vi "wsRegUnregEvents.vi"(8 "Error In":errorcluster, 9 "Event Name (empty =all)":string, 10 "Action":enum16{"Register", "Unregister"}(ring), 11 "References":T1) -> (0 "Error Out":errorcluster, 3 "References Out":T1)   [LabVIEW 2018, in "HASS-LV-WS_integration.lvlib"]
uses:
  HASS-LV-WS_integration.lvlib
  TypeDef/ReferencesTypeDef.ctl
  TypeDef/QueueTypeDef.ctl
  TypeDef/EventTypeDef.ctl
  TypeDef/registeredEventTypeDef.ctl
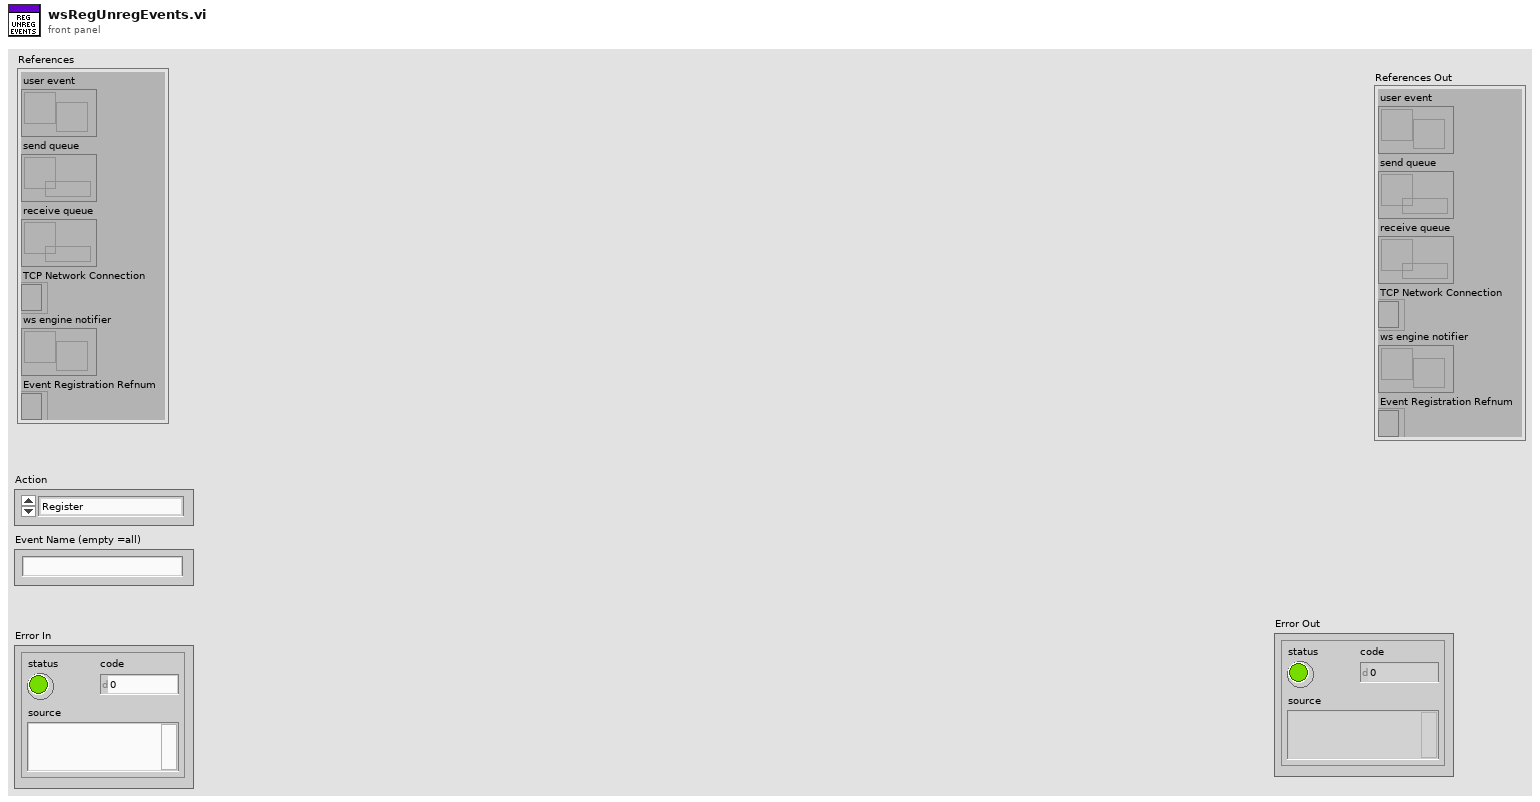
[diagram p1: front panel]
types:
  T1 = typedef "HASS-LV-WS_integration.lvlib/ReferencesTypeDef.ctl" = cluster{"user event":refnum<user-event>, "send queue":refnum<queue>, "receive queue":refnum<queue>, "TCP Network Connection":refnum<k5>, "ws engine notifier ":refnum<notifier>, "Event Registration Refnum":refnum<event-registration>}
  T2 = typedef "HASS-LV-WS_integration.lvlib/EventTypeDef.ctl" = cluster{"Data":variant, "Command":string}
  T3 = typedef "HASS-LV-WS_integration.lvlib/registeredEventTypeDef.ctl" = enum16{"Init", "Register", "Unregister", "Get MSG ID", "Get Event Name", "Get All Events"}
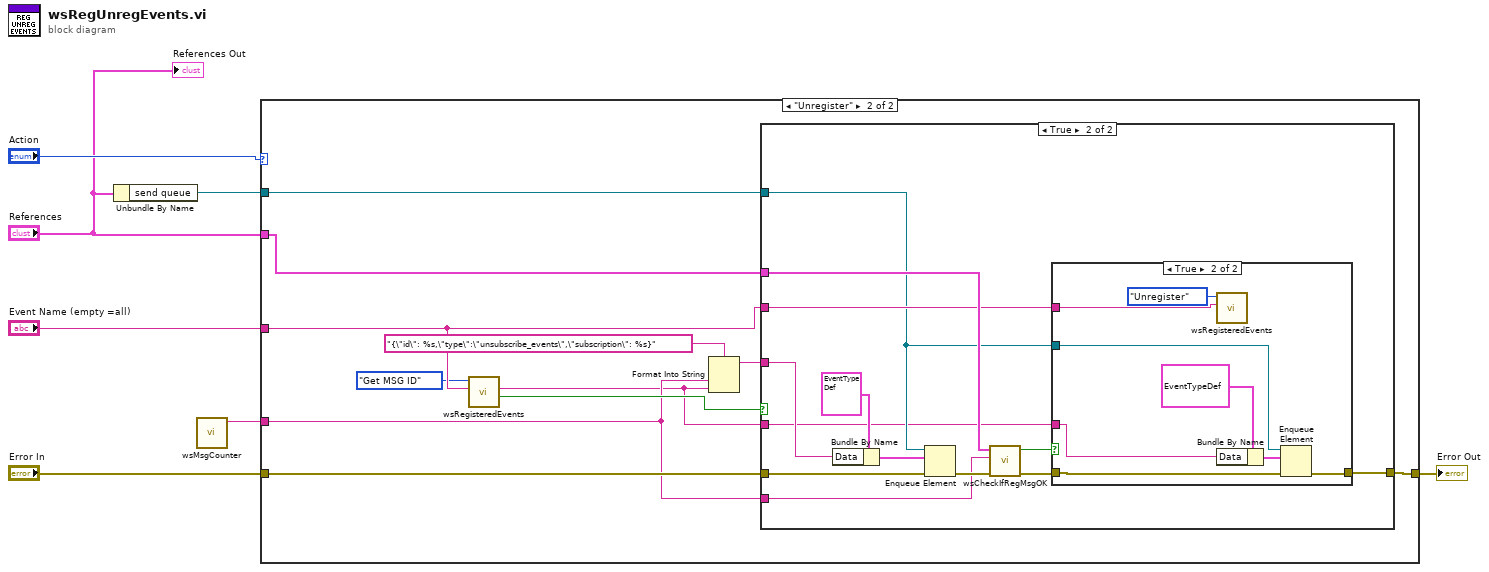
[diagram p0: block diagram]
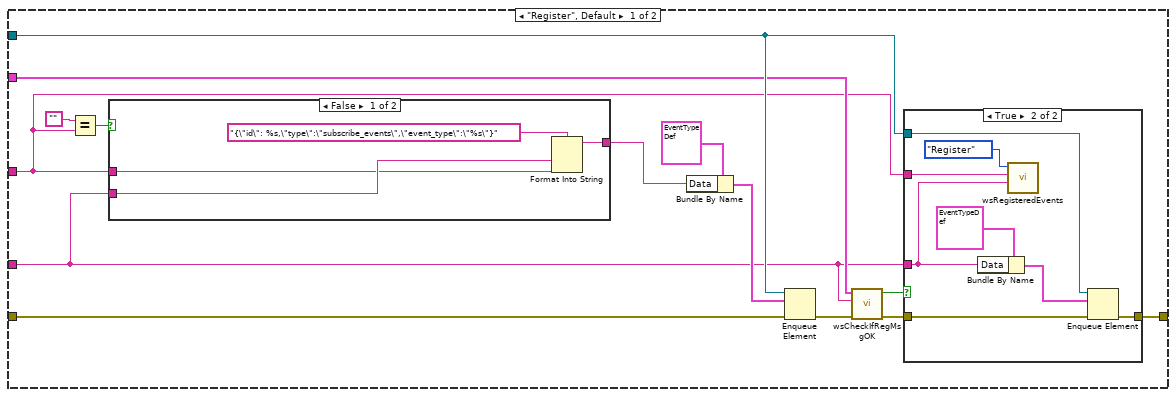
[diagram p2: hidden frame]
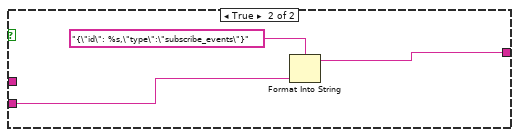
[diagram p4: hidden frame]
diagram:
  n1 = Unbundle By Name("References") -> ("send queue"=w6:refnum<queue>)
  n2 = call "wsMsgCounter.vi"() -> ("msgCounter"=w4:string)  [unwired: 11 in]
  n3 = case shown="\"Unregister\"" "Action" {
    tunnel: "Event Name (empty =all)" -> [w8 w42]
    tunnel: w4 -> [w9 w40]
    tunnel: w6 -> [w13 w46]
    tunnel: "Error In" -> [w16 w45]
    tunnel: "References" -> [w11 w43]
    tunnel: [w10 w41] -> w2
    frame "Register", Default {
      n4 = Equal?(x="", y=w8) -> (x = y?=w20:bool)
      n5 = case shown="False" w20 {
        tunnel: w9 -> [w33 w36]
        tunnel: w8 -> [w32 _]
        tunnel: [w31 w35] -> w17
        frame False {
          n6 = Format Into String(format string="{\"id\": %s,\"type\":\"subscribe_events\",\"event_type\":\"%s\"}", w33, w32) -> (resulting string=w31:string)  [unwired: 2 in, 1 out]
        }
        frame True {
          n7 = Format Into String(format string="{\"id\": %s,\"type\":\"subscribe_events\"}", w36) -> (resulting string=w35:string)  [unwired: 2 in, 1 out]
        }
      }
      n8 = Bundle By Name(cluster=T2 {"Data"=variant, "Command"="Send"} ("element"), "Data"=w17) -> (w18:T2)
      n9 = Enqueue Element(queue=w13, element=w18, error in (no error)=w16) -> (error out=w15:errorcluster)  [unwired: 1 in, 2 out]
      n10 = call "wsCheckIfRegMsgOK.vi"("error in (no error)"=w15, "msgCounter"=w9, "References"=w11) -> ("error out"=w12:errorcluster, "Success?"=w14:bool)  [unwired: 6 in, 1 out]
      n11 = case shown="True" w14 {
        tunnel: w9 -> [_ w26]
        tunnel: w8 -> [_ w30]
        tunnel: w13 -> [_ w29]
        tunnel: w12 -> [w22 w25]
        tunnel: [w22 w24] -> w10
        frame False {
        }
        frame True {
          n12 = Bundle By Name(cluster=T2 {"Data"=variant, "Command"="AddID"} ("element"), "Data"=w26) -> (w27:T2)
          n13 = call "wsRegisteredEvents.vi"("msgID"=w26, "Event Name (empty =all)"=w30, "Action"=registeredEventTypeDef."Register") -> ()  [unwired: 5 in, 4 out]
          n14 = Enqueue Element(queue=w29, element=w27, error in (no error)=w25) -> (error out=w24:errorcluster)  [unwired: 1 in, 2 out]
        }
      }
    }
    frame "Unregister" {
      n15 = call "wsRegisteredEvents.vi"("Event Name (empty =all)"=w42, "Action"=registeredEventTypeDef."Get MSG ID") -> ("Found?"=w47:bool, "Found ID"=w39:string)  [unwired: 6 in, 2 out]
      n16 = Format Into String(format string="{\"id\": %s,\"type\":\"unsubscribe_events\",\"subscription\": %s}", w40, w39) -> (resulting string=w44:string)  [unwired: 2 in, 1 out]
      n17 = case shown="True" w47 {
        tunnel: w46 -> [_ w53]
        tunnel: w45 -> [w49 w60]
        tunnel: [w49 w52] -> w41
        tunnel: w44 -> [_ w59]
        tunnel: w43 -> [_ w58]
        tunnel: w42 -> [_ w54]
        tunnel: w40 -> [_ w51]
        tunnel: w39 -> [_ w50]
        frame False {
        }
        frame True {
          n18 = Bundle By Name(cluster=T2 {"Data"=variant, "Command"="Send"} ("element"), "Data"=w59) -> (w61:T2)
          n19 = Enqueue Element(queue=w53, element=w61, error in (no error)=w60) -> (error out=w57:errorcluster)  [unwired: 1 in, 2 out]
          n20 = call "wsCheckIfRegMsgOK.vi"("error in (no error)"=w57, "msgCounter"=w51, "References"=w58) -> ("error out"=w55:errorcluster, "Success?"=w56:bool)  [unwired: 6 in, 1 out]
          n21 = case shown="True" w56 {
            tunnel: w55 -> [w63 w70]
            tunnel: [w63 w69] -> w52
            tunnel: w54 -> [_ w71]
            tunnel: w53 -> [_ w68]
            tunnel: w50 -> [_ w65]
            frame False {
            }
            frame True {
              n22 = call "wsRegisteredEvents.vi"("Event Name (empty =all)"=w71, "Action"=registeredEventTypeDef."Unregister") -> ()  [unwired: 6 in, 4 out]
              n23 = Bundle By Name(cluster=T2 {"Data"=variant, "Command"="RemoveID"} ("element"), "Data"=w65) -> (w66:T2)
              n24 = Enqueue Element(queue=w68, element=w66, error in (no error)=w70) -> (error out=w69:errorcluster)  [unwired: 1 in, 2 out]
            }
          }
        }
      }
    }
  }
  "Error Out" <- w2
  "References Out" <- "References"
